vi "Get Goal Coords From Map.vi"(1 "Coords":T1, 2 "CtlRef":refnum<vi>) -> (0 "Goal Coords":dbl[](array[numeric]))   [LabVIEW 2011]
uses:
  <vilib>/Utility/miscctls.llb/LVPoint32TypeDef.ctl
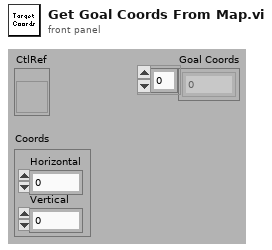
[diagram p1: front panel]
types:
  T1 = typedef "LVPoint32TypeDef.ctl" = cluster{"Horizontal":i32, "Vertical":i32}
  T2 = typedef "LVBoundsTypeDef.ctl" = cluster{"Width":u32, "Height":u32}
  T3 = typedef "LVPositionTypeDef.ctl" = cluster{"Left":i32, "Top":i32}
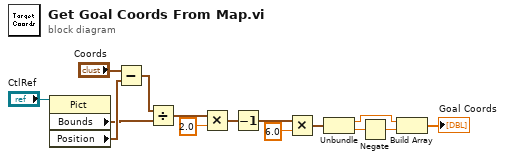
[diagram p0: block diagram]
diagram:
  n1 = property class="Pict"(reference="CtlRef") -> ("Bounds"=w3:T2, "Position"=w6:T3)  [unwired: 1 in, 2 out]
  n2 = Subtract(x="Coords", y=w6) -> (x-y=w8:T1)
  n3 = Divide(x=w8, y=w3) -> (x/y=w10:cluster{dbl, dbl})
  n4 = Multiply(x=w10, y=2.0) -> (x*y=w11:cluster{dbl, dbl})
  n5 = Decrement(x=w11) -> (x-1=w13:cluster{dbl, dbl})
  n6 = Multiply(x=w13, y=6.0) -> (x*y=w14:cluster{dbl, dbl})
  n7 = Unbundle(w14) -> (w4:dbl, w5:dbl)
  n8 = Negate(x=w5) -> (-x=w15:dbl)
  n9 = Build Array(w4, w15) -> (→"Goal Coords":dbl[])
